vi "Release Session.vi"(0 "Session Handle":T1, 11 "error in (no error)":errorcluster, 13 "force destroy? (F)":bool) -> (15 "error out":errorcluster)   [LabVIEW 2020, in "TSS.lvlib" / "Engine.lvclass"]
doc: "Releases an obtained reference to the session"
uses:
  Engine.lvclass
  Typedefs/Session Handle.ctl
  C:/Program Files (x86)/National Instruments/LabVIEW 2020/user.lib/_Session Fwk/Session - Root.lvclass
  <userlib>/_Session Fwk/Session - Root.lvclass
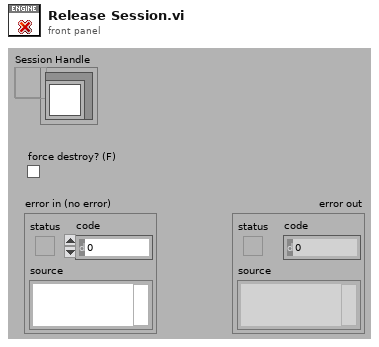
[diagram p1: front panel]
types:
  T1 = typedef "TSS.lvlib/Engine.lvclass/Session Handle.ctl" = refnum<data-value>
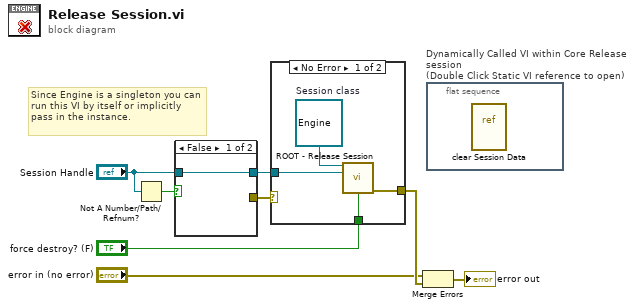
[diagram p0: block diagram]
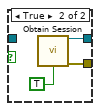
[diagram p2: hidden frame]
diagram:
  # "Since Engine is a singleton you can run this VI by itself or implicitly pass in the instance."
  n1 = Not A Number/Path/Refnum?(number/path/refnum="Session Handle") -> (NaN/Path/Refnum?=w6:bool)
  n2 = case shown="False" w6 {
    tunnel: "Session Handle" -> [w9 _]
    tunnel: [w9 w11] -> w4
    tunnel: [_ w10] -> w3
    frame False {
    }
    frame True {
      n3 = call "Obtain Session.vi"("Error to Create? (F)"=TRUE) -> ("Session Handle"=w11:T1, "error out"=w10:errorcluster)  [unwired: 13 in]
    }
  }
  n4 = case shown="No Error" w3 {
    selector: w3 -> [_ w17]
    tunnel: [w16 w17] -> w8
    tunnel: "force destroy? (F)" -> [w15 _]
    tunnel: w4 -> [w13 _]
    frame No Error {
      w14 = refnum<class "Engine.lvclass"> refnum  # Session class
      n5 = call <userlib>:"ROOT - Release Session.vi"("OBJ - Session in"=w14, "Session Handle in"=w13, "force destroy? (F)"=w15) -> ("error out"=w16:errorcluster)  [unwired: 11 in, 1 out]
    }
    frame Error {
    }
  }
  n6 = Merge Errors("error in (no error)", w8) -> (→"error out":errorcluster)
  n7 = flat-sequence "Dynamically Called VI within Core Release session\n(Double Click Static VI reference to open)" {
    frame #0 {
      n8 = vi-ref "clear Session Data.vi"() -> ()  [unwired: 1 out]
    }
  }
